vi "Check Packet Length.vi"(8 "error in (no error)":errorcluster, 10 "Mode":T1, 11 "payload in":u8[](array[numeric]) format="%.0x") -> (0 "error out":errorcluster, 3 "payload out":u8[](array[numeric]) format="%.0x")   [LabVIEW 2021, in "CAN_Logic.lvclass"]
uses:
  CAN_Logic.lvclass
  typedef/CAN Mode.ctl
  typedef/Error Global.vi
  CAN_Logic.lvclass/CAN_Logic.ctl
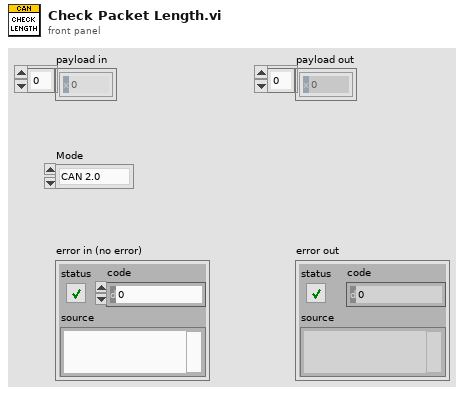
[diagram p1: front panel]
types:
  T1 = typedef "CAN_Logic.lvclass/CAN Mode.ctl" = enum16{"CAN 2.0", "CAN FD"}
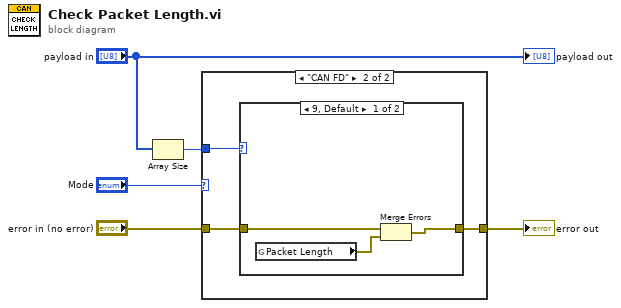
[diagram p0: block diagram]
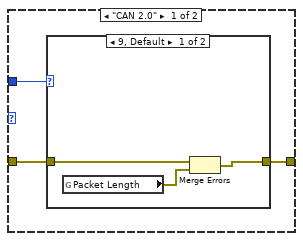
[diagram p2: hidden frame]
diagram:
  n1 = Array Size(array="payload in") -> (size(s)=w3:i32)
  n2 = case shown="\"CAN FD\"" "Mode" {
    tunnel: w3 -> [w8 w15]
    tunnel: "error in (no error)" -> [w7 w14]
    tunnel: [w6 w13] -> w1
    frame "CAN 2.0" {
      n3 = case shown="9, Default" w8 {
        tunnel: w7 -> [w11 w12]
        tunnel: [w9 w12] -> w6
        frame 9, Default {
          n4 = global read "Error Global.vi" "Packet Length"() -> (w10:errorcluster)
          n5 = Merge Errors(w11, w10) -> (w9:errorcluster)
        }
        frame 0..8 {
        }
      }
    }
    frame "CAN FD" {
      n6 = case shown="9, Default" w15 {
        tunnel: w14 -> [w18 w19]
        tunnel: [w16 w19] -> w13
        frame 9, Default {
          n7 = global read "Error Global.vi" "Packet Length"() -> (w17:errorcluster)
          n8 = Merge Errors(w18, w17) -> (w16:errorcluster)
        }
        frame 0..8, 12, 16, 20, 24, 32, 48, 64 {
        }
      }
    }
  }
  "error out" <- w1
  "payload out" <- "payload in"
